vi "Signal_averaging_diag.vi"(9 "Pike removed":cluster{"xi used":dbl[], "yi":dbl[]}(graph), 10 "Cutoff Frequency":dbl=500.0, 11 "Sampling Freq":dbl=5000.0) -> (2 "Averaged":cluster{"xi used":dbl[], "yi":dbl[]}(graph), 3 "Averaging window":dbl=10.0)   [LabVIEW 2015]
panel:
  out "averaged t":dbl[](array[numeric])
  out "averaged signal":dbl[](array[numeric])
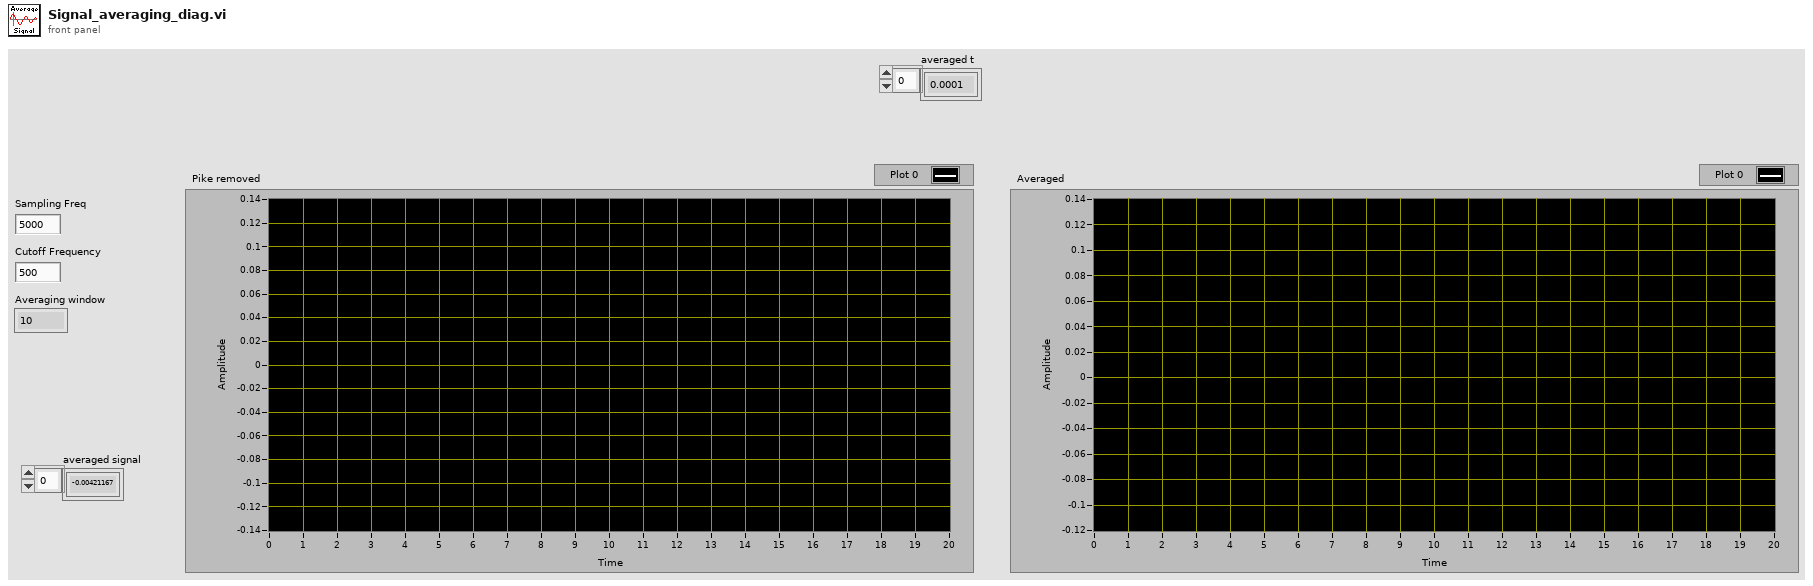
[diagram p1: front panel]
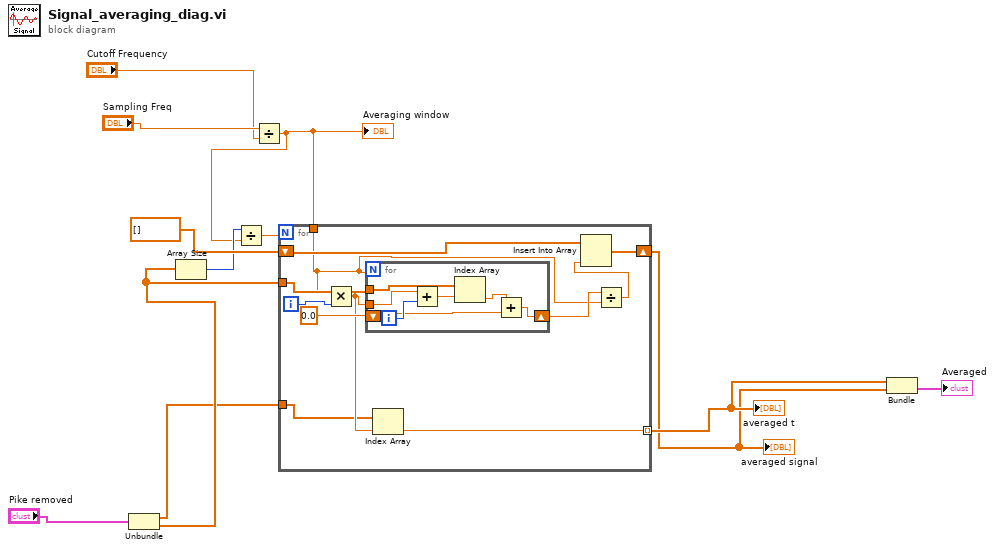
[diagram p0: block diagram]
diagram:
  n1 = Unbundle("Pike removed") -> ("xi used"=w4:dbl[], "yi"=w8:dbl[])
  n2 = Array Size(array=w8) -> (size(s)=w11:i32)
  n3 = Divide(x="Sampling Freq", y="Cutoff Frequency") -> (x/y=w5:dbl)
  "Averaging window" <- w5
  n4 = Divide(x=w11, y=w5) -> (x/y=w10:dbl)
  n5 = for {
    N: w10 -> [_]
    tunnel: w8 -> [w21]
    shift-right: [w22] -> w2
    shift-left: dbl[] [] -> [w23]
    tunnel: w5 -> [w16]
    tunnel: w4 -> [w14]
    tunnel: [w13] -> w3 mode=indexing
    i -> [w17]
    n6 = Multiply(x=w16, y=w17) -> (x*y=w15:dbl)
    n7 = for {
      N: w16 -> [_]
      tunnel: w21 -> [w30]
      tunnel: w15 -> [w28]
      shift-right: [w25] -> w20
      shift-left: 0.0 -> [w24]
      i -> [w27]
      n8 = Add(x=w28, y=w27) -> (x+y=w29:dbl)
      n9 = Index Array(array=w30, index=w29) -> (element=w26:dbl)
      n10 = Add(x=w26, y=w24) -> (x+y=w25:dbl)
    }
    n11 = Index Array(array=w14, index=w15) -> (element=w13:dbl)
    n12 = Divide(x=w20, y=w16) -> (x/y=w19:dbl)
    n13 = Insert Into Array(array=w23, new element=w19) -> (w22:dbl[])  [unwired: 1 in]
  }
  "averaged signal" <- w2
  "averaged t" <- w3
  n14 = Bundle(w3, w2) -> (→"Averaged":cluster{dbl[], dbl[]})  [unwired: 1 in]
